vi "statistics_test.vi"() -> ()   [LabVIEW 2018]
uses:
  <vilib>/Analysis/5stat.llb/RMS (DBL).vi
  <vilib>/Analysis/NI_AALBase.lvlib
  <vilib>/Analysis/NI_AALPro.lvlib
  <vilib>/gmath/NI_Gmath.lvlib
panel:
  in  "Number of factors":i32
  in  "type of design":T1(ring)
  out "XY 그래프":cluster{"X":dbl, "Y":dbl}[](graph)
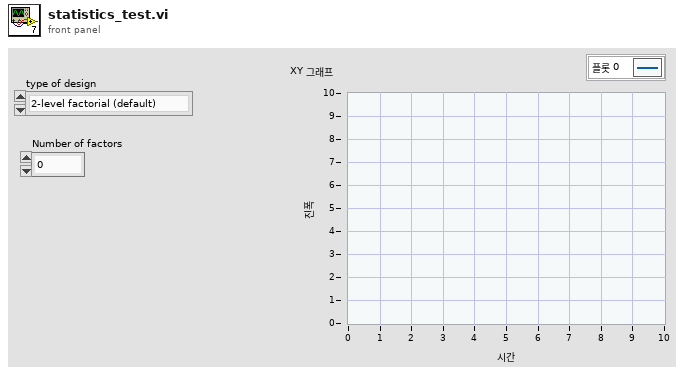
[diagram p1: front panel]
types:
  T1 = enum16{"2-level factorial (default)", "2-level factorial (specifiy)", "plackett-Burman design", "General full factorial design"}
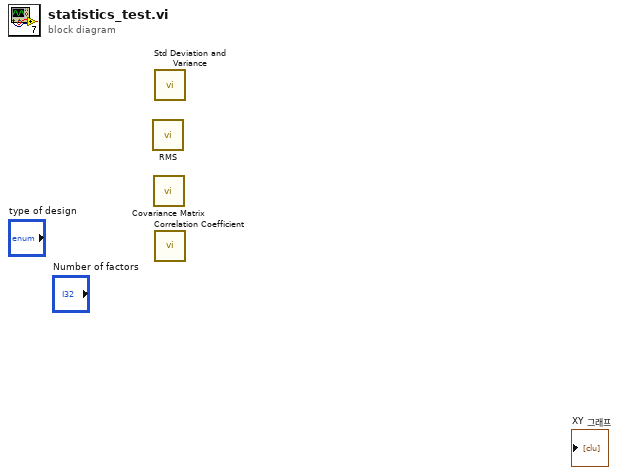
[diagram p0: block diagram]
diagram:
  n1 = call-poly <vilib>:"RMS.vi"() -> ()  [unwired: 1 in, 2 out]
  n2 = call <vilib>:"Covariance Matrix.vi"() -> ()  [unwired: 10 in, 2 out]
  n3 = call <vilib>:"Std Deviation and Variance.vi"() -> ()  [unwired: 2 in, 3 out]
  n4 = call <vilib>:"Correlation Coefficient.vi"() -> ()  [unwired: 10 in, 2 out]
